vi "Transfer Function (DBL).vi"(2 "initialize":bool, 3 "dt":dbl=1e-09 min=1e-09 format="%.6f", 4 "transfer function":cluster{"numerator":dbl[], "denominator":dbl[]} {"denominator" format="%.2f"; "numerator" format="%.2f"}, 5 "input point":dbl format="%.2f") -> (1 "output point":dbl format="%.2f")   [LabVIEW 2017, in "NI_AdvCtrl_continuous linear.lvlib"]
doc: "LabVIEW no longer supports this VI. You can obtain similar functionality by installing the LabVIEW Simulation Module.\n\nCalculates the new output point, where the transfer function and the input point are given. The transfer function is described by two polynomials, numerator and denominator."
uses:
  <vilib>/addons/control/advanced/NI_AdvCtrl_continuous linear.lvlib
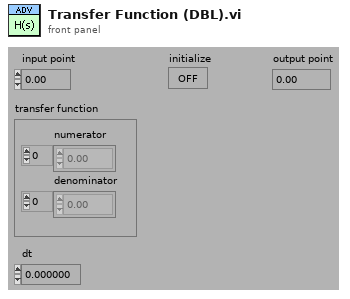
[diagram p1: front panel]
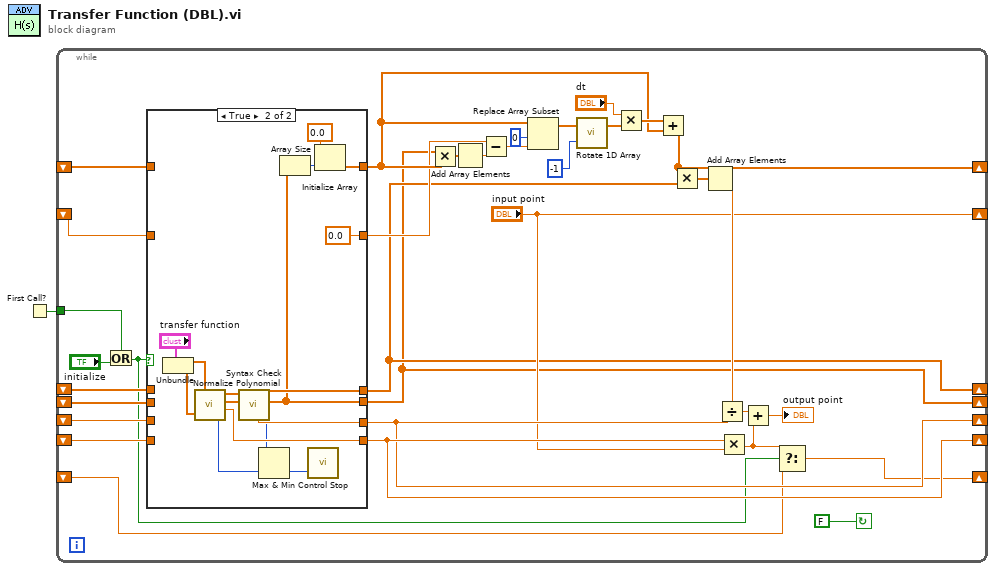
[diagram p0: block diagram]
diagram:
  n1 = First Call?() -> (First Call?: T/F=w1:bool)
  n2 = while {
    shift-left: _ -> [w16]
    shift-right: ["input point"] -> _
    shift-left: _ -> [w27]
    shift-right: [w20] -> _
    tunnel: w1 -> [w28]
    shift-left: _ -> [w7]
    shift-right: [w6] -> _
    shift-left: _ -> [w32]
    shift-right: [w31] -> _
    shift-left: _ -> [w33]
    shift-right: [w30] -> _
    shift-left: _ -> [w34]
    shift-right: [w12] -> _
    shift-left: _ -> [w35]
    shift-right: [w13] -> _
    stop <- FALSE continue-if-true
    n3 = Or(x=w28, y="initialize") -> (x .or. y?=w9:bool)
    n4 = case shown="True" w9 {
      tunnel: [w38 w57] -> w31
      tunnel: [w39 w50] -> w30
      tunnel: [w41 w54] -> w13
      tunnel: [w40 w46] -> w12
      tunnel: w35 -> [w41 _]
      tunnel: w34 -> [w40 _]
      tunnel: w33 -> [w39 _]
      tunnel: w32 -> [w38 _]
      tunnel: [w37 w44] -> w19
      tunnel: w27 -> [w37 _]
      tunnel: [w36 0.0 ("input point")] -> w15
      tunnel: w16 -> [w36 _]
      frame False {
      }
      frame True {
        n5 = Unbundle("transfer function") -> ("numerator"=w52:dbl[], "denominator"=w47:dbl[])
        n6 = call <vilib>:"Normalize Polynomial.vi"("Numerator"=w52, "Denominator"=w47) -> ("Numerator new"=w55:dbl[], "Denominator new"=w56:dbl[], "additive constant"=w57:dbl, "error"=w48:i32)
        n7 = call <vilib>:"Syntax Check.vi"("Denominator"=w56, "Numerator"=w55) -> ("error"=w49:i32, "gain"=w50:dbl, "Denominator new"=w46:dbl[], "Numerator new"=w54:dbl[])  [unwired: 1 out]
        n8 = Max & Min(x=w49, y=w48) -> (min(x,y)=w42:i32)  [unwired: 1 out]
        n9 = Array Size(array=w46) -> (size(s)=w45:i32)
        n10 = call <vilib>:"Control Stop.vi"("error"=w42) -> ()  [unwired: 2 out]
        n11 = Initialize Array(0.0, w45) -> (w44:dbl[])
      }
    }
    n12 = Multiply(x=w12, y=w19) -> (x*y=w24:dbl[])
    n13 = Add Array Elements(numeric array=w24) -> (sum=w23:dbl)
    n14 = Subtract(x=w15, y=w23) -> (x-y=w26:dbl)
    n15 = Replace Array Subset(array=w19, new element=w26, index=0 ("Index")) -> (w5:dbl[])
    n16 = call <vilib>:"Rotate 1D Array.vi"("n"=-1, "array"=w5) -> ("array (last n elements first)"=w4:dbl[])  [unwired: 1 out]
    n17 = Multiply(x="dt", y=w4) -> (x*y=w22:dbl[])
    n18 = Add(x=w22, y=w19) -> (x+y=w20:dbl[])
    n19 = Multiply(x=w20, y=w13) -> (x*y=w21:dbl[])
    n20 = Add Array Elements(numeric array=w21) -> (sum=w18:dbl)
    n21 = Divide(x=w18, y=w30) -> (x/y=w11:dbl)
    n22 = Multiply(x=w31, y="input point") -> (x*y=w8:dbl)
    n23 = Add(x=w11, y=w8) -> (x+y=→"output point":dbl)
    n24 = Select(t=w8, s=w9, f=w7) -> (s? t:f=w6:dbl)
  }
